vi "Post Build Action Edited.vi"(5 "Files Generated by Build":path[](array[path]), 6 "Top Level/Always Included VIs":path[](array[path]), 7 "Destination Path":path, 8 "error in (no error)":errorcluster, 9 "Target Name":string, 10 "Build Specification Name":string, 11 "Project Path":path) -> (0 "error out":errorcluster)   [LabVIEW 2018, in "Support Library.lvlib"]
uses:
  Support Library.lvlib
  <vilib>/Utility/sysdir.llb/System Directory Type.ctl
  <vilib>/Utility/config.llb/Write Key (Boolean).vi
  <vilib>/Utility/config.llb/Write Key (Path).vi
  <vilib>/Utility/config.llb/Write Key (String).vi
  <vilib>/Utility/config.llb/NI_LVConfig.lvlib
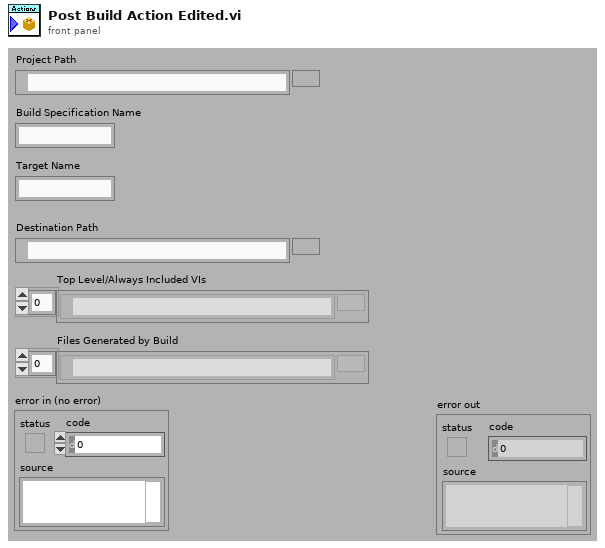
[diagram p1: front panel]
types:
  T1 = typedef "System Directory Type.ctl" = i32
  T2 = typedef "NI_LVConfig.lvlib/Config Data RefNum.ctl" = refnum<k1>
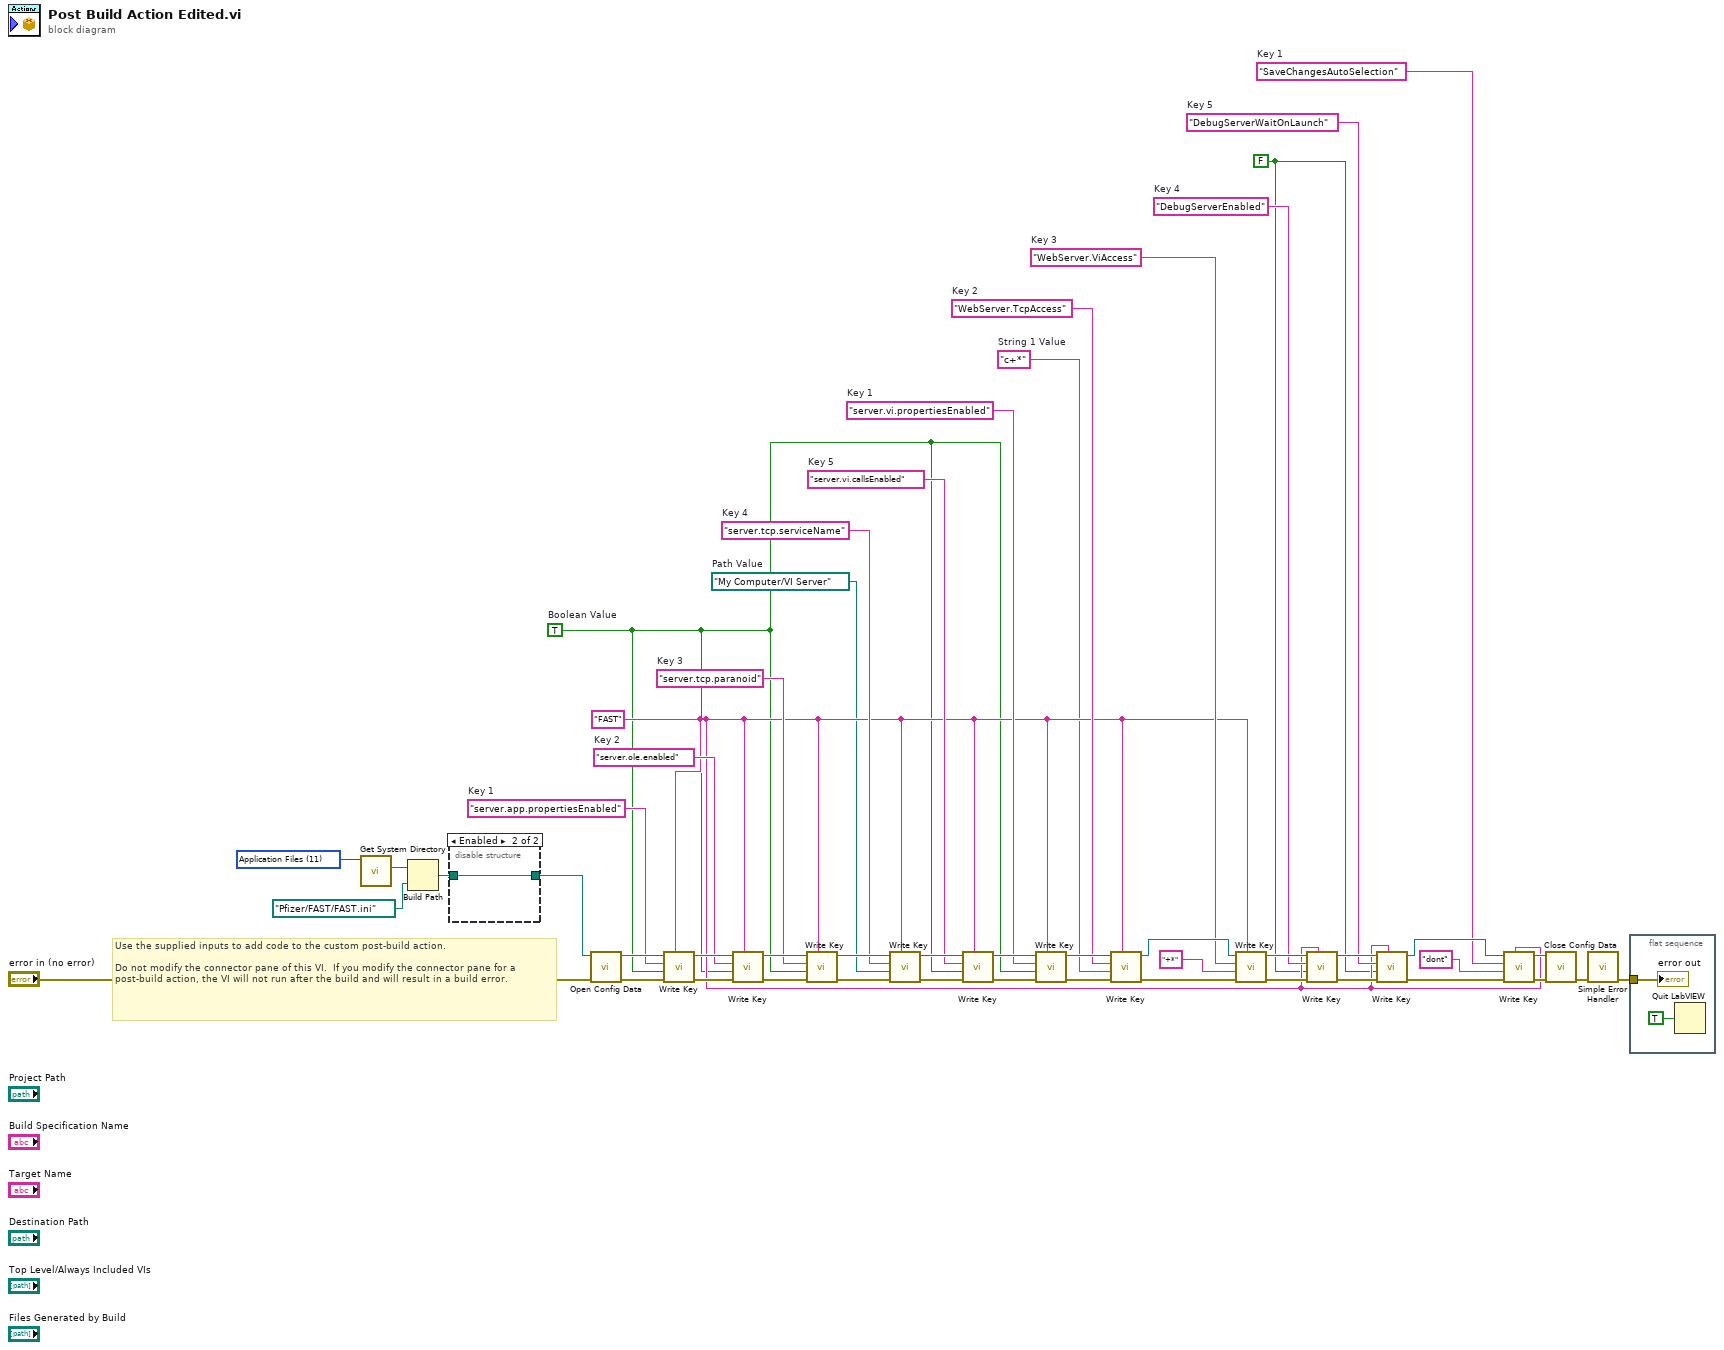
[diagram p0: block diagram]
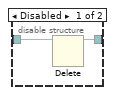
[diagram p2: hidden frame]
diagram:
  w3 = T1 11 items=["User Home"=0, "User Desktop"=1, "User Documents"=2, "User Application Data"=3, "User Preferences"=4, "User Temporary"=5, "Public Documents"=6, "Public Application Data"=7, "Public Preferences"=8, "Public Cache"=13, "System Core Libraries"=9, "System Installed Libraries"=10, "Application Files"=11, "Boot Volume Root"=12] ("system directory type")
  w8 = FALSE ("value")
  w14 = "SaveChangesAutoSelection"  # Key 1
  w15 = "DebugServerWaitOnLaunch"  # Key 5
  w16 = "DebugServerEnabled"  # Key 4
  w17 = "WebServer.ViAccess"  # Key 3
  w18 = "WebServer.TcpAccess"  # Key 2
  w19 = "server.vi.propertiesEnabled"  # Key 1
  w10 = "c+*"  # String 1 Value
  w12 = path "My Computer/VI Server"  # Path Value
  w11 = TRUE  # Boolean Value
  w36 = "server.vi.callsEnabled"  # Key 5
  w37 = "server.tcp.serviceName"  # Key 4
  w38 = "server.tcp.paranoid"  # Key 3
  w39 = "server.ole.enabled"  # Key 2
  w40 = "server.app.propertiesEnabled"  # Key 1
  w13 = "FAST"
  # "Use the supplied inputs to add code to the custom post-build action.\n\nDo not modify the connector pane of this VI.  If you modify the connector pane for a post-build action, the VI will not run after the build and will result in a build error."
  n1 = call <vilib>:"Get System Directory.vi"("system directory type"=w3) -> ("system directory"=w5:path)  [unwired: 10 in]
  n2 = Build Path(base path=w5, name or relative path=path "Pfizer/FAST/FAST.ini" ("default name")) -> (appended path=w4:path)
  n3 = disable-structure shown="Enabled" {
    disable-tunnel: [w52 w53] -> w34
    disable-tunnel: w4 -> [w51 w53]
    frame Disabled {
      n4 = Delete(path (use dialog)=w51) -> (deleted path=w52:path)  [unwired: 4 in, 2 out]
    }
    frame Enabled {
    }
  }
  n5 = call <vilib>:"Open Config Data.vi"("error in (no error)"="error in (no error)", "configuration file path"=w34) -> ("error out"=w45:errorcluster, "refnum"=w50:T2)  [unwired: 1 in, 7 out]
  n6 = call-poly <vilib>:"Write Key.vi"("section"=w13, "error in (no error)"=w45, "value"=w11, "key"=w40, "refnum"=w50) -> ("error out"=w44:errorcluster, "refnum out"=w49:T2)  [unwired: 5 out]
  n7 = call-poly <vilib>:"Write Key.vi"("section"=w13, "error in (no error)"=w44, "value"=w11, "key"=w39, "refnum"=w49) -> ("error out"=w43:errorcluster, "refnum out"=w48:T2)  [unwired: 5 out]
  n8 = call-poly <vilib>:"Write Key.vi"("section"=w13, "error in (no error)"=w43, "value"=w11, "key"=w38, "refnum"=w48) -> ("error out"=w42:errorcluster, "refnum out"=w47:T2)  [unwired: 5 out]
  n9 = call-poly <vilib>:"Write Key.vi"("section"=w13, "error in (no error)"=w42, "value"=w12, "key"=w37, "refnum"=w47) -> ("error out"=w41:errorcluster, "refnum out"=w46:T2)  [unwired: 1 in, 4 out]
  n10 = call-poly <vilib>:"Write Key.vi"("section"=w13, "error in (no error)"=w41, "value"=w11, "key"=w36, "refnum"=w46) -> ("error out"=w21:errorcluster, "refnum out"=w20:T2)  [unwired: 1 in, 4 out]
  n11 = call-poly <vilib>:"Write Key.vi"("section"=w13, "error in (no error)"=w21, "value"=w11, "key"=w19, "refnum"=w20) -> ("error out"=w30:errorcluster, "refnum out"=w26:T2)  [unwired: 5 out]
  n12 = call-poly <vilib>:"Write Key.vi"("section"=w13, "error in (no error)"=w30, "value"=w10, "key"=w18, "refnum"=w26) -> ("error out"=w31:errorcluster, "refnum out"=w27:T2)  [unwired: 1 in, 4 out]
  n13 = call-poly <vilib>:"Write Key.vi"("section"=w13, "error in (no error)"=w31, "value"="+*", "key"=w17, "refnum"=w27) -> ("error out"=w32:errorcluster, "refnum out"=w28:T2)  [unwired: 1 in, 4 out]
  n14 = call-poly <vilib>:"Write Key.vi"("section"=w13, "error in (no error)"=w32, "value"=w8, "key"=w16, "refnum"=w28) -> ("error out"=w33:errorcluster, "refnum out"=w29:T2)  [unwired: 1 in, 4 out]
  n15 = call-poly <vilib>:"Write Key.vi"("section"=w13, "error in (no error)"=w33, "value"=w8, "key"=w15, "refnum"=w29) -> ("error out"=w23:errorcluster, "refnum out"=w22:T2)  [unwired: 1 in, 4 out]
  n16 = call-poly <vilib>:"Write Key.vi"("section"=w13, "error in (no error)"=w23, "value"="dont", "key"=w14, "refnum"=w22) -> ("error out"=w24:errorcluster, "refnum out"=w25:T2)  [unwired: 1 in, 4 out]
  n17 = call <vilib>:"Close Config Data.vi"("error in (no error)"=w24, "refnum"=w25) -> ("error out"=w35:errorcluster)  [unwired: 1 in, 8 out]
  n18 = call <vilib>:"Simple Error Handler.vi"("error in (no error)"=w35) -> ("error out"=w1:errorcluster)  [unwired: 1 in, 7 out]
  n19 = flat-sequence {
    tunnel: w1 -> [w55]
    frame #0 {
      n20 = Quit LabVIEW(quit? (T)=TRUE) -> ()
      "error out" <- w55
    }
  }
